vi "Unflatten XML String.vi"(8 "Error In":errorcluster, 10 "XML String":string, 11 "Tree Manager":T1) -> (0 "Error Out":errorcluster, 3 "Tree Manager":T1)   [LabVIEW 2016, in "Tree Manager.lvclass"]
doc: "Load the XML String specification of the Tree structure. \n\n<b>WARNING</b> When using this on an already existing Tree multiple Roots will be defined. Use the List Roots method to select the appropriate one for further use. To make sure only the contents of the XML will be represented in the resulting Tree obtain a new empty reference before calling this method."
uses:
  Tree Manager.lvclass
  Typedefs/Session Handle.ctl
  Tree Manager.lvclass/Tree Manager.ctl
  <vilib>/xml/Close Reference(Node).vi
  <vilib>/xml/NI_XML.lvlib
  <resource>/objmgr/DOMUserDefRef.rc
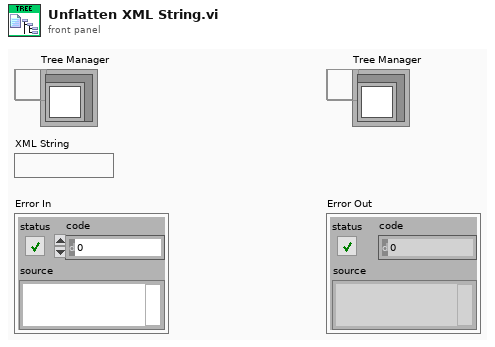
[diagram p1: front panel]
types:
  T1 = typedef "Tree Manager.lvclass/Session Handle.ctl" = refnum<data-value>
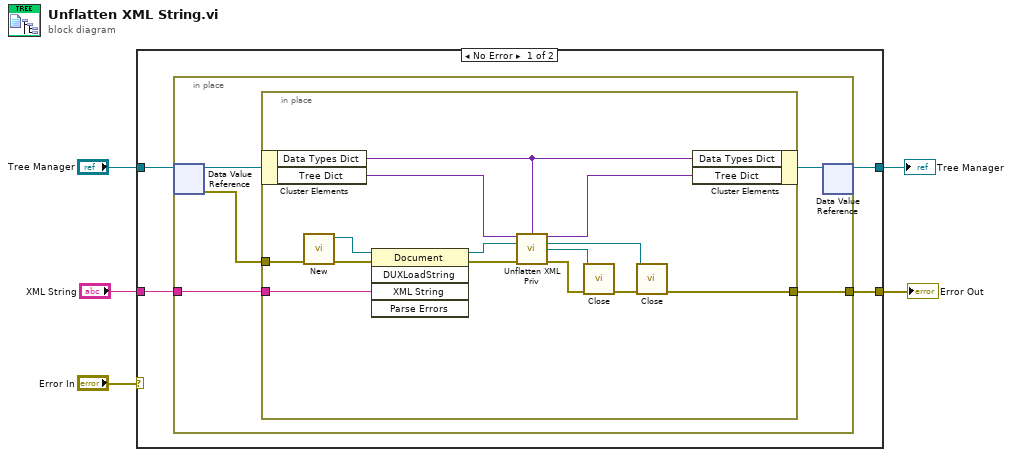
[diagram p0: block diagram]
diagram:
  n1 = case shown="No Error" "Error In" {
    selector: "Error In" -> [_ w29]
    tunnel: "Tree Manager" -> [w9 w30]
    tunnel: [w8 w30] -> w4
    tunnel: [w6 w29] -> w2
    tunnel: "XML String" -> [w7 _]
    frame No Error {
      n2 = in-place {
        in-place-border: w7 -> [w12]
        in-place-border: [w11] -> w6
        n3 = in-place-dvr #1(w9) -> (w14:refnum<class "Tree Manager.lvclass">, w10:errorcluster)
        n4 = in-place {
          in-place-border: w12 -> [w22]
          in-place-border: [w15] -> w11
          in-place-border: w10 -> [w25]
          n5 = in-place-cluster #2(w14) -> ("Data Types Dict"=w27:variant, "Tree Dict"=w26:variant)
          n6 = call <vilib>:"New.vi"("error in (no error)"=w25) -> ("error out"=w24:errorcluster, "DOM document out"=w23:refnum<k20>)  [unwired: 7 in]
          n7 = invoke class="Document" method="DUXLoadString"(reference=w23, error in=w24, "XML String"=w22) -> (reference out=w21:refnum<k20>, error out=w20:errorcluster)  [unwired: 2 in, 3 out]
          n8 = call "Unflatten XML Priv.vi"("Tree Dict in"=w26, "Data Types Dict"=w27, "DOM Doc In"=w21, "Error In"=w20) -> ("Tree Dict out"=w28:variant, "DOM Doc Out"=w16:refnum<k20>, "Parent Element"=w18:refnum<k20>, "Error Out"=w19:errorcluster)  [unwired: 8 in]
          n9 = call-poly <vilib>:"Close.vi"("error in (no error)"=w19, "node"=w18) -> ("error out"=w17:errorcluster)  [unwired: 7 in]
          n10 = call-poly <vilib>:"Close.vi"("error in (no error)"=w17, "node"=w16) -> ("error out"=w15:errorcluster)  [unwired: 7 in]
          n11 = in-place-cluster #2("Data Types Dict"=w27, "Tree Dict"=w28) -> (w13:refnum<class "Tree Manager.lvclass">)
        }
        n12 = in-place-dvr #1(w13) -> (w8:T1)  [unwired: 1 out]
      }
    }
    frame Error {
    }
  }
  "Tree Manager" <- w4
  "Error Out" <- w2
